vi "Clear ListView.vi"(8 "error in (no error)":errorcluster caption="错误输入（无错误）", 11 "ListViewClass 输入":refnum<class "ListViewClass.lvclass"> caption="DNL_LabVIEW Object in") -> (0 "error out":errorcluster caption="错误输出", 3 "ListViewClass 输出":refnum<class "ListViewClass.lvclass"> caption="DNL_LabVIEW Object out")   [LabVIEW 2012, in "ListViewClass.lvclass"]
uses:
  ListViewClass.lvclass
  ListViewClass.lvclass/ListViewClass.ctl
  System.Windows.Forms
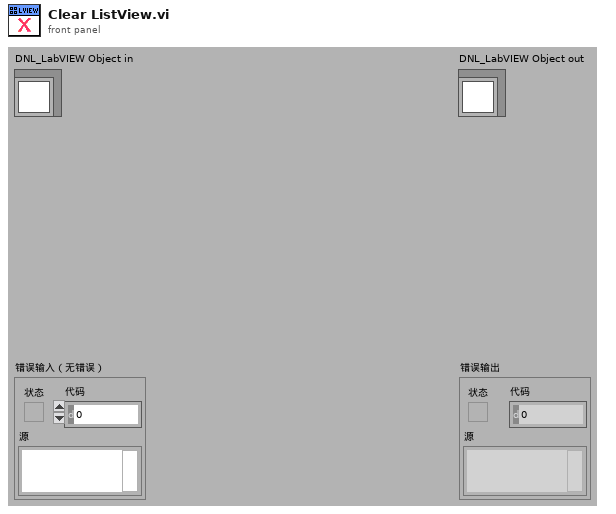
[diagram p1: front panel]
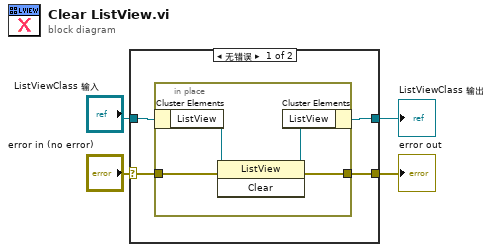
[diagram p0: block diagram]
diagram:
  n1 = case shown="无错误" "error in (no error)" {
    selector: "error in (no error)" -> [w7 w14]
    tunnel: [w6 w14] -> w3
    tunnel: [w5 w13] -> w1
    tunnel: "ListViewClass 输入" -> [w8 w13]
    frame No Error {
      n2 = in-place {
        in-place-border: w7 -> [w10]
        in-place-border: [w9] -> w6
        n3 = in-place-cluster #1(w8) -> ("ListView"=w12:refnum<k24>)
        n4 = invoke class="ListView" method="Clear"(reference=w12, error in=w10) -> (reference out=w11:refnum<k24>, error out=w9:errorcluster)  [unwired: 1 in, 1 out]
        n5 = in-place-cluster #1("ListView"=w11) -> (w5:refnum<class "ListViewClass.lvclass">)
      }
    }
    frame Error {
    }
  }
  "error out" <- w3
  "ListViewClass 输出" <- w1
